vi "testIntAdd.vi"(8 "error in (no error)":errorcluster, 11 "TestCase in":refnum<class "UnitTestIntClass.lvclass">) -> (0 "error out":errorcluster, 3 "TestCase out":refnum<class "UnitTestIntClass.lvclass">)   [LabVIEW 2011, in "UnitTestIntClass.lvclass"]
uses:
  UnitTestIntClass.lvclass
  UnitTestIntClass.lvclass/UnitTestIntClass.ctl
  <vilib>/addons/_JKI Toolkits/VI Tester/TestCase.llb/TestCase.lvclass
  IntClass/IntClass.lvclass
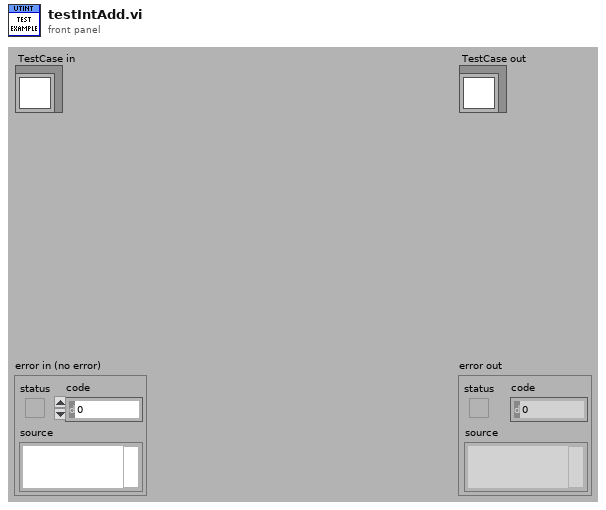
[diagram p1: front panel]
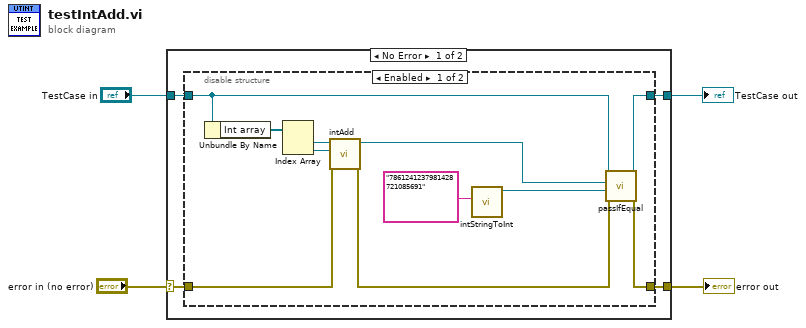
[diagram p0: block diagram]
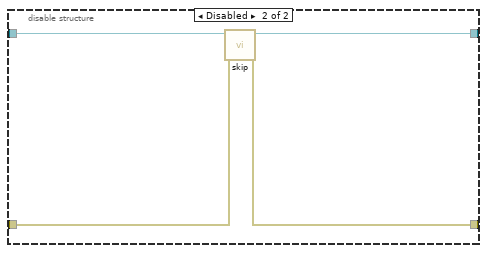
[diagram p2: hidden frame]
diagram:
  n1 = case shown="No Error" "error in (no error)" {
    selector: "error in (no error)" -> [w6 w25]
    tunnel: [w5 w25] -> w3
    tunnel: [w7 w24] -> w1
    tunnel: "TestCase in" -> [w8 w24]
    frame No Error {
      n2 = disable-structure shown="Enabled" {
        disable-tunnel: w8 -> [w17 w23]
        disable-tunnel: [w19 w20] -> w7
        disable-tunnel: w6 -> [w15 w22]
        disable-tunnel: [w18 w21] -> w5
        frame Enabled {
          n3 = Unbundle By Name(w17) -> ("Int array"=w16:refnum<class "IntClass.lvclass">[])
          n4 = Index Array(array=w16) -> (element #1=w10:refnum<class "IntClass.lvclass">, element #2=w9:refnum<class "IntClass.lvclass">)  [unwired: 2 in]
          n5 = call "intAdd.vi"("Error in (no error)"=w15, "Int2 in"=w9, "Int1 in"=w10) -> ("Error out"=w14:errorcluster, "Int1 + Int2"=w13:refnum<class "IntClass.lvclass">)  [unwired: 6 in, 1 out]
          n6 = call "intStringToInt.vi"("String in"="7861241237981428721085691") -> ("Int out"=w11:refnum<class "IntClass.lvclass">)  [unwired: 9 in, 1 out]
          n7 = call-dynamic "passIfEqual.vi"("error in (no error)"=w14, "y"=w11, "x"=w13, "TestCase in"=w17) -> ("error out"=w18:errorcluster, "TestCase out"=w19:refnum<class "UnitTestIntClass.lvclass">)  [unwired: 6 in]
        }
        frame Disabled {
          n8 = call <vilib>:"skip.vi"("error in (no error)"=w22, "TestCase in"=w23) -> ("error out"=w21:errorcluster, "TestCase out"=w20:refnum<class "UnitTestIntClass.lvclass">)  [unwired: 8 in]
        }
      }
    }
    frame Error {
    }
  }
  "error out" <- w3
  "TestCase out" <- w1
